vi "Write WaitKick.vi"(8 "error in (no error)":errorcluster, 10 "WaitKick":bool, 11 "KickToSkill in":refnum<class "KickToSkill.lvclass">) -> (0 "error out":errorcluster, 3 "KickToSkill out":refnum<class "KickToSkill.lvclass">)   [LabVIEW 2023, in "KickToSkill.lvclass"]
uses:
  KickToSkill.lvclass
  KickToSkill.lvclass/KickToSkill.ctl
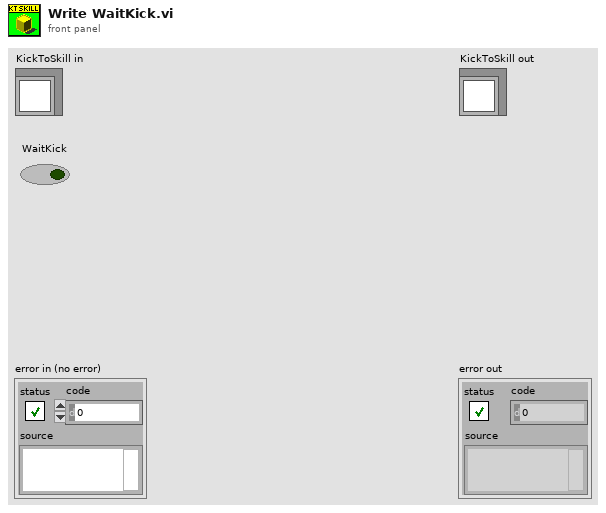
[diagram p1: front panel]
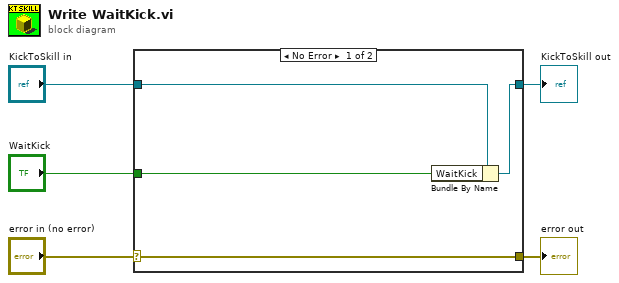
[diagram p0: block diagram]
diagram:
  n1 = case shown="No Error" "error in (no error)" {
    selector: "error in (no error)" -> [w9 w10]
    tunnel: [w9 w10] -> w4
    tunnel: [w7 w11] -> w2
    tunnel: "KickToSkill in" -> [w8 w11]
    tunnel: "WaitKick" -> [w6 _]
    frame No Error {
      n2 = Bundle By Name(cluster=w8, "WaitKick"=w6) -> (w7:refnum<class "KickToSkill.lvclass">)
    }
    frame Error {
    }
  }
  "error out" <- w4
  "KickToSkill out" <- w2
